vi "Write.vi"(6 "Mask payload?":bool, 7 "Opcode (Text)":T1=1 items=["Cont. Frame"=0, "Text"=1, "Binary"=2, "Ping"=9, "Pong"=10], 8 "error in (no error)":errorcluster, 9 "timeout ms (5000)":i32=5000, 10 "Data":string, 11 "WebSocket Connection in":refnum<k5>) -> (0 "error out":errorcluster, 3 "WebSocket Connection out":refnum<k5>)   [LabVIEW 2013, in "WebSockets.lvlib"]
doc: "Sends a WebSocket message to the client. Messages sent from the client must be masked but it is optional for the server.\n\nFinished should be set to True unless sending a fragmented message."
uses:
  WebSockets.lvlib
  Opcodes.ctl
panel:
  in  "Finished? (True)":bool=TRUE
  # "(leave as 'True' unless sending fragmented messages)"
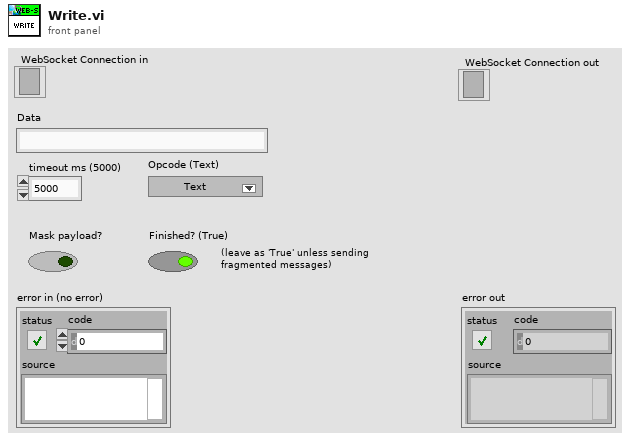
[diagram p1: front panel]
types:
  T1 = typedef "WebSockets.lvlib/Opcodes.ctl" = u8
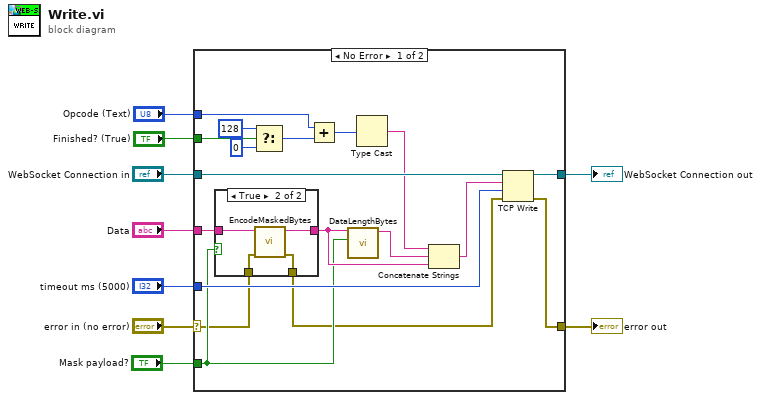
[diagram p0: block diagram]
diagram:
  n1 = case shown="No Error" "error in (no error)" {
    selector: "error in (no error)" -> [w17 w35]
    tunnel: [w25 w35] -> w8
    tunnel: [w27 w34] -> w6
    tunnel: "WebSocket Connection in" -> [w26 w34]
    tunnel: "Data" -> [w20 _]
    tunnel: "timeout ms (5000)" -> [w21 _]
    tunnel: "Mask payload?" -> [w18 _]
    tunnel: "Finished? (True)" -> [w15 _]
    tunnel: "Opcode (Text)" -> [w12 _]
    frame No Error {
      n2 = case shown="True" w18 {
        tunnel: w20 -> [w29 w33]
        tunnel: [w29 w32] -> w19
        tunnel: w17 -> [w28 w31]
        tunnel: [w28 w30] -> w16
        frame False {
        }
        frame True {
          n3 = call "EncodeMaskedBytes.vi"("error in (no error)"=w31, "Raw Data"=w33) -> ("error out"=w30:errorcluster, "Encoded Data"=w32:string)  [unwired: 8 in]
        }
      }
      n4 = Select(t=u8 128, s=w15, f=u8 0) -> (s? t:f=w13:u8)
      n5 = Add(x=w12, y=w13) -> (x+y=w14:T1)
      n6 = call "DataLengthBytes.vi"("Is masked?"=w18, "Data"=w19) -> ("Length Bytes"=w24:string)  [unwired: 9 in]
      n7 = Type Cast(x=w14) -> (*(type *) &x=w23:string)  [unwired: 1 in]
      n8 = Concatenate Strings(w23, w24, w19) -> (w22:string)
      n9 = TCP Write(connection ID=w26, data in=w22, error in (no error)=w16, 9:w21) -> (connection ID out=w27:refnum<k5>, error out=w25:errorcluster)  [unwired: 1 out]
    }
    frame Error {
    }
  }
  "WebSocket Connection out" <- w6
  "error out" <- w8
